vi "Motion Profile Tester.vi"() -> ()   [LabVIEW 2015]
uses:
  <vilib>/Rock Robotics/WPI/CAN/TalonSRX/WPI_CANTalonSRX_MotionProfileTrajectoryPt.ctl
  <vilib>/Rock Robotics/WPI/CAN/TalonSRX/WPI_CANTalonSRX_APIControlMode.ctl
  <vilib>/Rock Robotics/WPI/CAN/TalonSRX/WPI_CANTalonSRX_APIFeedbackSelect.ctl
  <vilib>/Rock Robotics/WPI/MotorControl/WPI_MotorControlOpenCANTalonSRX.vi
panel:
  in  "Generate, Load, and Run Profile":bool
  in  "Run Profile":bool
  in  "Load Profile":bool
  in  "Generate Profile and Clear Points":bool
  out "XY Graph":cluster{dbl[], dbl[]}[](graph)
  in  "Mode":T1(ring)
  in  "Motion Profile Control Frame Rate":dbl
  in  "Rotations to Travel":dbl
  in  "Max Jerk (rotations/sec^3)":dbl
  in  "Max Acceleration (rotations/sec^2)":dbl
  in  "Max Speed (rotations/sec)":dbl
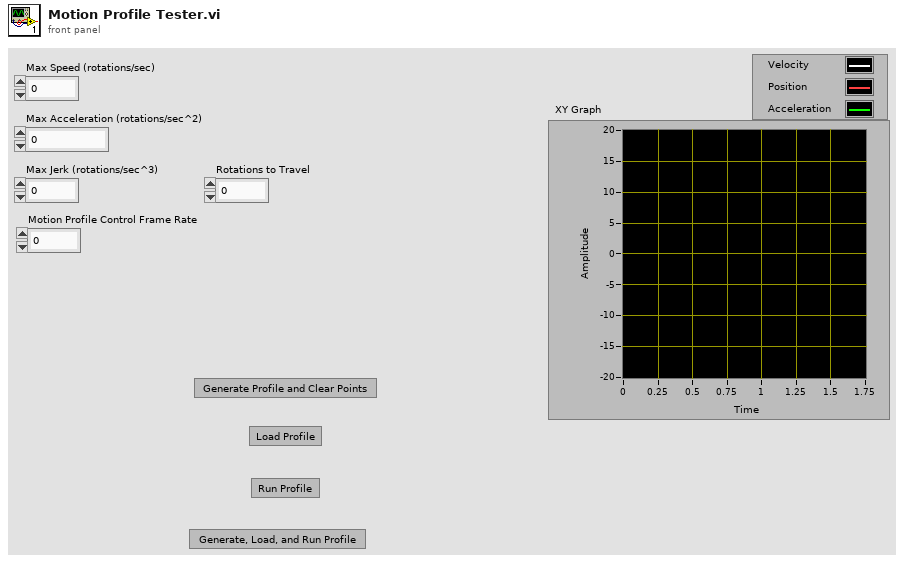
[diagram p1: front panel]
types:
  T1 = enum16{"Nothing", "Generate Profile and Clear", "Load Data to Motor", "Run Profile"}
  T2 = typedef "WPI_CANTalonSRX_APIFeedbackSelect.ctl" = enum16{"Digital Quadrature Encoder", "Analog Potentiometer", "Analog Encoder", "Count on Quad-A (Rising-Edge)", "Count on Quad-A (Falling-Edge)", "CTR Magnetic Enc (Absolute)", "CTR Magnetic Enc (Relative)", "Pulse Width"}
  T3 = typedef "WPI_CANTalonSRX_APIControlMode.ctl" = enum8{"Percent VBus", "Speed", "Position", "Slave", "Unchanged / Invalid", "Voltage Compensation", "Current", "Motion Profile"}
  T4 = typedef "WPI_MotorControlDeviceRef.ctl" = cluster{"DeviceStatus":errorcluster, "Type":T5, "PWM":cluster{"PWM Channel":T6, "DeadBand":T7}, "CAN":cluster{"Device Number":u8, "Control Mode":T8, "Semaphore":T9, "Max Vout":dbl, "TalonSRX Control Mode":T3}, "Invert":bool}
  T5 = typedef "WPI_MotorControlType.ctl" = enum16{"PWM", "CAN", "CANTalonSRX"}
  T6 = typedef "FPGA_DIOPWMChannel.ctl" = enum8{"PWM 0", "PWM 1", "PWM 2", "PWM 3", "PWM 4", "PWM 5", "PWM 6", "PWM 7", "PWM 8", "PWM 9", "PWM MXP 0", "PWM MXP 1", "PWM MXP 2", "PWM MXP 3", "PWM MXP 4", "PWM MXP 5", "PWM MXP 6", "PWM MXP 7", "PWM MXP 8", "PWM MXP 9", "Invalid"}
  T7 = typedef "WPI_PWMDeadband.ctl" = cluster{"Name":string, "maxPositivePwm":i32, "minPositivePwm":i32, "centerPwm":i32, "maxNegativePwm":i32, "minNegativePwm":i32, "angularRange":u16}
  T8 = typedef "WPI_CANJaguar_ControlMode.ctl" = enum8{"Percent VBus", "Current", "Speed", "Position", "Voltage"}
  T9 = typedef "Semaphore RefNum" = refnum<k1>
  T10 = typedef "WPI_CANTalonSRX_MotionProfileTrajectoryPt.ctl" = cluster{"Duration Ms":u8, "Velocity":dbl, "Position":dbl, "Profile Slot Select":u8, "Is Last":bool, "Velocity Only":bool, "Zero Position":bool, "Compress Code":u8, "Same Velocity":i32, "Delta Position":i32, "Count":u8}
  T11 = enum16{"Nothing", "Generate Profile and Clear", "Load Data to Motor", "Run Profile"}[]
  T12 = typedef "WPI_CANTalonSRX_GlobalStatus.ctl" = cluster{"Applied Throttle":dbl, "Module Enabled":bool, "CAN Error":errorcluster, "Closed Loop Error":dbl, "Forward Limit Switch Closed":bool, "Reverse Limit Switch Closed":bool, "Sensor Position":dbl, "Sensor Velocity":dbl, "Current":dbl, "Sticky Fault - Over Temp":bool, "Sticky Fault - Under Voltage":bool, "Sticky Fault - Forward Limit":bool, "Sticky Fault - Reverse Limit":bool, "Sticky Fault - Forward Soft Limit":bool, "Sticky Fault - Reverse Soft Limit":bool, "Brake is Enabled":bool, "Encoder Position":dbl, "Encoder Velocity":dbl, "Encoder Index Count":dbl, "Encoder A Pin State":bool, "Encoder B Pin State":bool, "Encoder Index Pin State":bool, "Analog In":dbl, "Analog In Velocity":dbl, "Temperature (C)":dbl, "Battery Voltage":dbl, "Control 5 Is Supported":bool, "Current Profile Slot Select":dbl, "Pos Div 8":bool, "Vel Div 4":bool, "Pulse Width Position":i32, "Pulse Width Velocity":i32, "Pulse Width Rise To Rise (us)":i32, "Pulse Width Rise To Fall (us)":i32, "Mot Prof Active Is Under Run":bool, "Mot Prof Active Has Under Run":bool, "Mot Prof Active Is Last":bool, "Mot Prof Active Velocity Only":bool, "Mot Prof Active Is Valid":bool, "Mot Prof Buffer Is Full":bool, "Mot Prof Active Profile Slot Select":i32, "Mot Prof NextID":i32, "Mot Prof Count":i32, "Mot Prof Active Velocity":dbl, "Mot Prof Active Position":dbl, "Mot Prof Output Enable":i32}
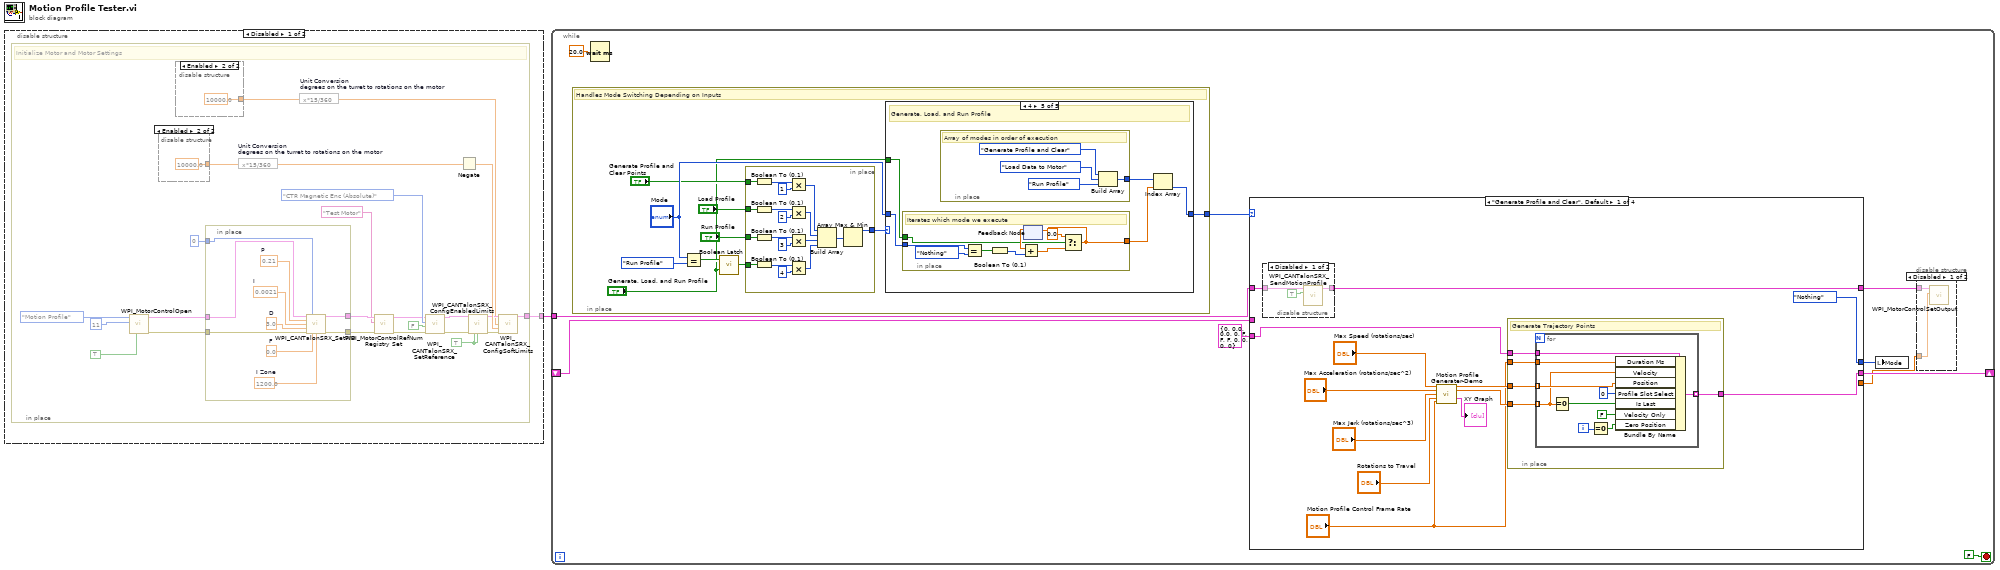
[diagram p0: block diagram]
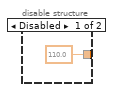
[diagram p2: hidden frame]
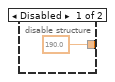
[diagram p3: hidden frame]
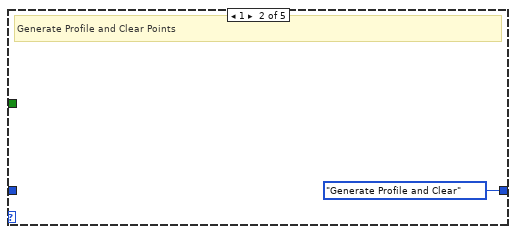
[diagram p6: hidden frame]
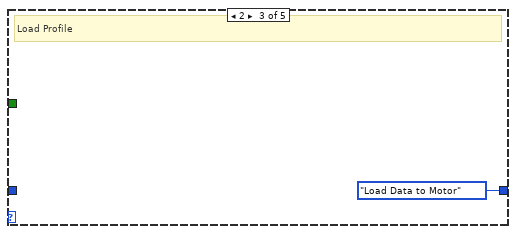
[diagram p7: hidden frame]
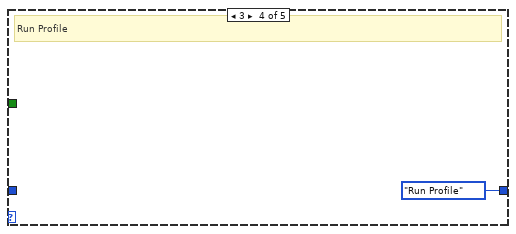
[diagram p8: hidden frame]
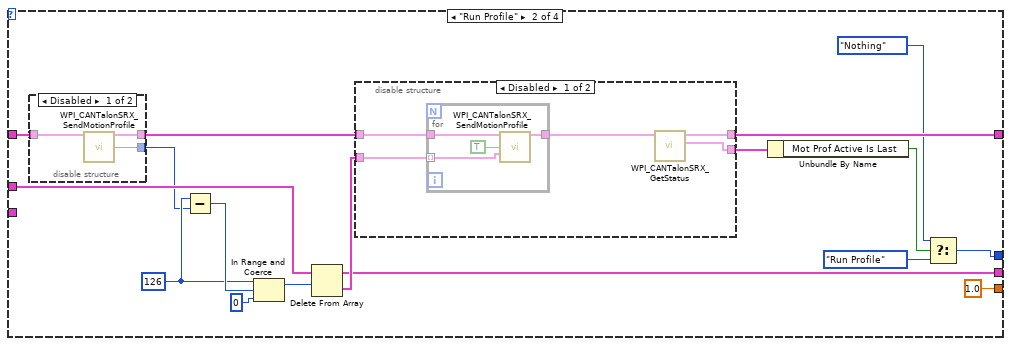
[diagram p11: hidden frame]
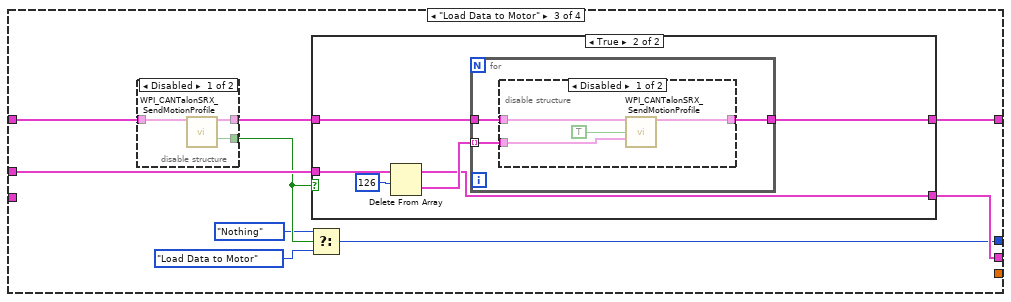
[diagram p14: hidden frame]
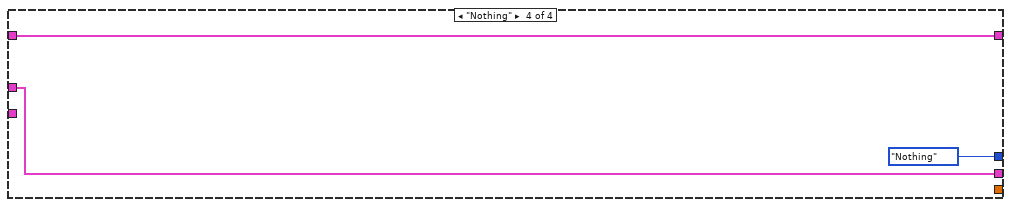
[diagram p18: hidden frame]
diagram:
  n1 = disable-structure shown="Disabled" {
    disable-tunnel: [w2 _] -> w1
    frame Disabled {
      n2 = in-place {
        in-place-border: [w20] -> w2
        w16 = TRUE ("Forward Soft Limit Enable")
        # "Initialize Motor and Motor Settings"
        n3 = call-poly <vilib>:"WPI_MotorControlOpen.vi"("Invert"=TRUE, "Device Number"=11, "Control Mode"=WPI_CANTalonSRX_APIControlMode."Motion Profile") -> ("error out"=w23:errorcluster, "MotorControlDeviceRef"=w24:T4)  [unwired: 7 in]
        n4 = disable-structure shown="Enabled" {
          disable-tunnel: [110.0 ("Forward Limit Position") 10000.0 ("Forward Limit Position")] -> w19
          frame Disabled {
          }
          frame Enabled {
          }
        }
        n5 = disable-structure shown="Enabled" {
          disable-tunnel: [190.0 ("Forward Limit Position") 10000.0 ("Forward Limit Position")] -> w11
          frame Disabled {
          }
          frame Enabled {
          }
        }
        n6 = in-place {
          in-place-border: w24 -> [w40]
          in-place-border: w23 -> [w39]
          in-place-border: [w31] -> w7
          in-place-border: [w32] -> w9
          in-place-border: u8 0 ("Parameter Slot") -> [w33]
          w34 = 1200.0  # I Zone
          w35 = 0.0  # F
          w36 = 3.0  # D
          w37 = 0.0021  # I
          w38 = 0.21  # P
          n7 = call <vilib>:"WPI_CANTalonSRX_SetPID.vi"("CAN Talon SRX Ref"=w40, "Parameter Slot"=w33, "P"=w38, "I"=w37, "D"=w36, "error in (no error)"=w39, "F"=w35, "I Zone"=w34) -> ("CAN Talon SRX Ref"=w32:T4, "error out"=w31:errorcluster)  [unwired: 6 in]
        }
        n8 = expression code="x*15/360" "Unit Conversion\ndegrees on the turret to rotations on the motor"(w19) -> (w18:dbl)
        n9 = expression code="x*15/360" "Unit Conversion\ndegrees on the turret to rotations on the motor"(w11) -> (w10:dbl)
        n10 = call <vilib>:"WPI_MotorControlRefNum Registry Set.vi"("error in (no error)"=w7, "refnum name"="Test Motor", "MotorControlDevRef"=w9) -> ("error out"=w6:errorcluster, "MotorControlDevRef"=w8:T4)  [unwired: 7 in]
        n11 = call <vilib>:"WPI_CANTalonSRX_SetReference.vi"("error in (no error)"=w6, "Reverse Feedback Sensor"=FALSE, "Feedback Reference"=WPI_CANTalonSRX_APIFeedbackSelect."CTR Magnetic Enc (Absolute)", "CAN Talon SRX Ref"=w8) -> ("error out"=w3:errorcluster, "CAN Talon SRX Ref"=w4:T4)  [unwired: 6 in]
        n12 = Negate(x=w18) -> (-x=w17:dbl)
        n13 = call <vilib>:"WPI_CANTalonSRX_ConfigEnabledLimits.vi"("CAN Talon SRX Ref"=w4, "error in (no error)"=w3, "Forward Soft Limit Enable"=w16, "Reverse Soft Limit Enable"=w16) -> ("CAN Talon SRX Ref"=w14:T4, "error out"=w15:errorcluster)  [unwired: 10 in]
        n14 = call <vilib>:"WPI_CANTalonSRX_ConfigSoftLimits.vi"("CAN Talon SRX Ref"=w14, "Forward Limit Position"=w10, "Reverse Limit Position"=w17, "error in (no error)"=w15) -> ("CAN Talon SRX Ref"=w20:T4)  [unwired: 10 in, 1 out]
      }
    }
    frame Enabled {
    }
  }
  n15 = while {
    tunnel: w1 -> [w50]
    shift-right: [w48] -> _
    shift-left: _ -> [w45]
    stop <- FALSE stop-if-true
    n16 = in-place {
      in-place-border: [w58] -> w41
      # "Handles Mode Switching Depending on Inputs"
      n17 = Equal?(x="Mode", y=T1."Run Profile") -> (x = y?=w59:bool)
      n18 = call "Boolean Latch.vi"("Input"="Generate, Load, and Run Profile", "Reset"=w59) -> ("Output"=w52:bool)
      n19 = in-place {
        in-place-border: "Generate Profile and Clear Points" -> [w78]
        in-place-border: "Load Profile" -> [w73]
        in-place-border: w52 -> [w71]
        in-place-border: "Run Profile" -> [w69]
        in-place-border: [w63] -> w54
        n20 = Boolean To (0,1)(Boolean=w78) -> (0, 1=w77:i16)
        n21 = Boolean To (0,1)(Boolean=w73) -> (0, 1=w75:i16)
        n22 = Boolean To (0,1)(Boolean=w69) -> (0, 1=w62:i16)
        n23 = Boolean To (0,1)(Boolean=w71) -> (0, 1=w61:i16)
        n24 = Multiply(x=w77, y=i16 1) -> (x*y=w68:i16)
        n25 = Multiply(x=w75, y=i16 2) -> (x*y=w67:i16)
        n26 = Multiply(x=w62, y=i16 3) -> (x*y=w66:i16)
        n27 = Multiply(x=w61, y=i16 4) -> (x*y=w65:i16)
        n28 = Build Array(w68, w67, w66, w65) -> (w64:i16[])
        n29 = Array Max & Min(array=w64) -> (max value=w63:i16)  [unwired: 3 out]
      }
      n30 = case shown="4" w54 {
        tunnel: [w79 T1."Generate Profile and Clear" ("Mode") T1."Load Data to Motor" ("Mode") T1."Run Profile" ("Mode") w83] -> w58
        tunnel: "Mode" -> [w79 _ _ _ w87]
        tunnel: "Generate, Load, and Run Profile" -> [_ _ _ _ w86]
        frame 0, Default {
          # "Carry last operation"
        }
        frame 1 {
          # "Generate Profile and Clear Points"
        }
        frame 2 {
          # "Load Profile"
        }
        frame 3 {
          # "Run Profile"
        }
        frame 4 {
          # "Generate, Load, and Run Profile"
          n31 = in-place {
            in-place-border: w87 -> [w96]
            in-place-border: w86 -> [w91]
            in-place-border: [w88] -> w84
            # "Iterates which mode we execute"
            n32 = Equal?(x=w96, y=T1."Nothing") -> (x = y?=w94:bool)
            n33 = Boolean To (0,1)(Boolean=w94) -> (0, 1=w93:i16)
            n34 = feedback #1() -> (w92:dbl)  [unwired: 1 in]
            n35 = Add(x=w92, y=w93) -> (x+y=w89:dbl)
            n36 = Select(t=0.0, s=w91, f=w89) -> (s? t:f=w88:dbl)
            n37 = feedback-in #1(w88) -> ()
          }
          n38 = in-place {
            in-place-border: [w97] -> w85
            # "Array of modes in order of execution"
            n39 = Build Array(T1."Generate Profile and Clear" ("y"), T1."Load Data to Motor" ("y"), T1."Run Profile" ("y")) -> (w97:T11)
          }
          n40 = Index Array(array=w85, index=w84) -> (element=w83:T1)
        }
      }
    }
    n41 = Wait (ms)(milliseconds to wait=20.0) -> ()  [unwired: 1 out]
    n42 = case shown="\"Generate Profile and Clear\", Default" w41 {
      tunnel: w50 -> [w111 w148 w170 w192]
      tunnel: T10 {"Duration Ms"=0, "Velocity"=0.0, "Position"=0.0, "Profile Slot Select"=0, "Is Last"=FALSE, "Velocity Only"=FALSE, "Zero Position"=FALSE, "Compress Code"=0, "Same Velocity"=0, "Delta Position"=0, "Count"=0} ("New Point") -> [w110 _ _ _]
      tunnel: [w106 w142 w168 w190] -> w48
      tunnel: [T1."Nothing" ("Mode") w139 w164 T1."Nothing" ("Mode")] -> w46
      tunnel: w45 -> [_ w149 w171 w190]
      tunnel: [w104 w141 w163 w192] -> w43
      tunnel: [_ 1.0 _ _] -> w42
      frame "Generate Profile and Clear", Default {
        n43 = disable-structure shown="Disabled" {
          disable-tunnel: w111 -> [w132 _]
          disable-tunnel: [w131 _] -> w104
          frame Disabled {
            n44 = call <vilib>:"WPI_CANTalonSRX_SendMotionProfile.vi"("CAN Talon SRX Ref"=w132, "Clear"=TRUE) -> ("CAN Talon SRX Ref Out"=w131:T4)  [unwired: 10 in, 3 out]
          }
          frame Enabled {
          }
        }
        n45 = call "Motion Profile Generater-Demo.vi"("Max Speed (rotations/sec)"="Max Speed (rotations/sec)", "Max Acceleration (rotations/sec^2)"="Max Acceleration (rotations/sec^2)", "Max Jerk (rotations/sec^3)"="Max Jerk (rotations/sec^3)", "Rotations to Travel"="Rotations to Travel", "Motion Profile Control Frame Rate"="Motion Profile Control Frame Rate") -> ("Position rotations"=w108:dbl[], "velocity rotations/sec"=w109:dbl[], "XY Graph"=→"XY Graph":cluster{dbl[], dbl[]}[])  [unwired: 7 in, 1 out]
        n46 = in-place {
          in-place-border: w110 -> [w120]
          in-place-border: w109 -> [w119]
          in-place-border: w108 -> [w118]
          in-place-border: "Motion Profile Control Frame Rate" -> [w117]
          in-place-border: [w116] -> w106
          # "Generate Trajectory Points"
          n47 = for {
            tunnel: w120 -> [w130]
            tunnel: w119 -> [w126] mode=indexing
            tunnel: w118 -> [w128] mode=indexing
            tunnel: w117 -> [w127]
            tunnel: [w121] -> w116 mode=indexing
            i -> [w123]
            n48 = Equal To 0?(x=w126) -> (x = 0?=w125:bool)
            n49 = Equal To 0?(x=w123) -> (x = 0?=w122:bool)
            n50 = Bundle By Name(cluster=w130, "Duration Ms"=w127, "Velocity"=w126, "Position"=w128, "Profile Slot Select"=u8 0, "Is Last"=w125, "Velocity Only"=FALSE, "Zero Position"=w122) -> (w121:T10)
          }
        }
      }
      frame "Run Profile" {
        w146 = u32 126 ("x")
        n51 = disable-structure shown="Disabled" {
          disable-tunnel: w148 -> [w162 _]
          disable-tunnel: [w161 _] -> w135
          disable-tunnel: [w160 _] -> w134
          frame Disabled {
            n52 = call <vilib>:"WPI_CANTalonSRX_SendMotionProfile.vi"("CAN Talon SRX Ref"=w162) -> ("CAN Talon SRX Ref Out"=w160:T4, "Count"=w161:u32)  [unwired: 11 in, 2 out]
          }
          frame Enabled {
          }
        }
        n53 = Subtract(x=w146, y=w135) -> (x-y=w147:u32)
        n54 = In Range and Coerce(upper limit=w146, x=w147, lower limit=u32 0) -> (coerced(x)=w143:u32)  [unwired: 1 out]
        n55 = Delete From Array(array=w149, length=w143) -> (deleted portion=w144:T10[], array with subset deleted=w142:T10[])  [unwired: 1 in]
        n56 = disable-structure shown="Disabled" {
          disable-tunnel: w144 -> [w155 _]
          disable-tunnel: [w154 _] -> w141
          disable-tunnel: [w153 _] -> w140
          disable-tunnel: w134 -> [w152 _]
          frame Disabled {
            n57 = for {
              tunnel: w155 -> [w159] mode=indexing
              tunnel: w152 -> [w157]
              tunnel: [w156] -> w151
              n58 = call <vilib>:"WPI_CANTalonSRX_SendMotionProfile.vi"("CAN Talon SRX Ref"=w157, "Push"=TRUE, "New Point"=w159) -> ("CAN Talon SRX Ref Out"=w156:T4)  [unwired: 9 in, 3 out]
            }
            n59 = call <vilib>:"WPI_CANTalonSRX_GetStatus.vi"("CAN Talon SRX Ref"=w151) -> ("Talon SRX Status"=w153:T12, "CAN Talon SRX Ref"=w154:T4)  [unwired: 8 in, 1 out]
          }
          frame Enabled {
          }
        }
        n60 = Unbundle By Name(w140) -> ("Mot Prof Active Is Last"=w138:bool)
        n61 = Select(t=T1."Nothing" ("Mode"), s=w138, f=T1."Run Profile" ("Mode")) -> (s? t:f=w139:T1)
      }
      frame "Load Data to Motor" {
        n62 = disable-structure shown="Disabled" {
          disable-tunnel: w170 -> [w174 _]
          disable-tunnel: [w173 _] -> w169
          disable-tunnel: [w172 _] -> w167
          frame Disabled {
            n63 = call <vilib>:"WPI_CANTalonSRX_SendMotionProfile.vi"("CAN Talon SRX Ref"=w174) -> ("CAN Talon SRX Ref Out"=w173:T4, "Ready For Next"=w172:bool)  [unwired: 11 in, 2 out]
          }
          frame Enabled {
          }
        }
        n64 = Select(t=T1."Nothing" ("Mode"), s=w167, f=T1."Load Data to Motor" ("Mode")) -> (s? t:f=w164:T1)
        n65 = case shown="True" w167 {
          tunnel: w171 -> [w176 w182]
          tunnel: w169 -> [w175 w179]
          tunnel: [w176 w178] -> w168
          tunnel: [w175 w177] -> w163
          frame False {
          }
          frame True {
            n66 = Delete From Array(array=w182, length=126) -> (deleted portion=w180:T10[], array with subset deleted=w178:T10[])  [unwired: 1 in]
            n67 = for {
              tunnel: w180 -> [w185] mode=indexing
              tunnel: w179 -> [w184]
              tunnel: [w183] -> w177
              n68 = disable-structure shown="Disabled" {
                disable-tunnel: w185 -> [w189 _]
                disable-tunnel: w184 -> [w188 _]
                disable-tunnel: [w186 _] -> w183
                frame Disabled {
                  n69 = call <vilib>:"WPI_CANTalonSRX_SendMotionProfile.vi"("CAN Talon SRX Ref"=w188, "Push"=TRUE, "New Point"=w189) -> ("CAN Talon SRX Ref Out"=w186:T4)  [unwired: 9 in, 3 out]
                }
                frame Enabled {
                }
              }
            }
          }
        }
      }
      frame "Nothing" {
      }
    }
    n70 = local write "Mode"(w46) -> ()
    n71 = disable-structure shown="Disabled" {
      disable-tunnel: w43 -> [w102 _]
      disable-tunnel: w42 -> [w101 _]
      frame Disabled {
        n72 = call <vilib>:"WPI_MotorControlSetOutput.vi"("Output"=w101, "MotorControlDevRef"=w102) -> ()  [unwired: 7 in, 3 out]
      }
      frame Enabled {
      }
    }
  }
